vi "SUB-module-문자열 파일 저장.vi"(4 "파일 경로":string, 5 "문자열":string) -> ()   [LabVIEW 2014]
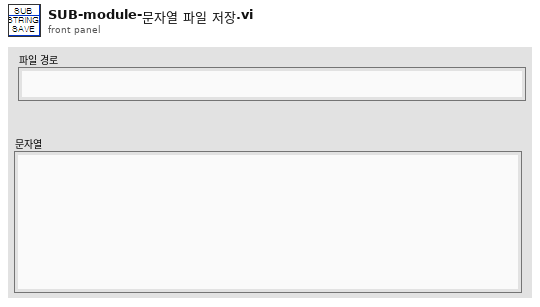
[diagram p1: front panel]
types:
  T1 = enum16{"open", "replace", "create", "open or create", "replace or create", "replace or create with confirmation"}
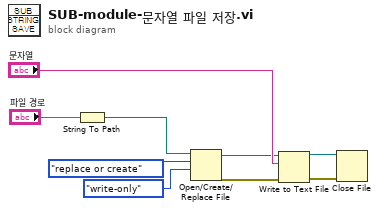
[diagram p0: block diagram]
diagram:
  n1 = String To Path(string="파일 경로") -> (path=w1:path)
  n2 = Open/Create/Replace File(file path (use dialog)=w1, operation (0:open)=T1."replace or create" ("동작(0:open)"), access (0:read/write)=enum16{"read/write", "read-only", "write-only"}."write-only" ("접근(0:읽기/쓰기)")) -> (refnum out=w7:refnum<file>, error out=w8:errorcluster)  [unwired: 1 in, 3 out]
  n3 = Write to Text File(file (use dialog)=w7, text="문자열", error in=w8) -> (refnum out=w6:refnum<file>, error out=w5:errorcluster)  [unwired: 2 out]
  n4 = Close File(refnum=w6, error in=w5) -> ()  [unwired: 2 out]
